vi "Set Time Context.vi"(0 "Tree in":refnum<class "Tree.lvclass">, 5 "Start":refnum<class "Data.lvclass">, 7 "End":refnum<class "Data.lvclass">, 9 "Delta":refnum<class "Data.lvclass">, 11 "error in (no error)":errorcluster) -> (4 "Tree out":refnum<class "Tree.lvclass">, 15 "error out":errorcluster)   [LabVIEW 2012, in "MDSplus.lvlib" / "Tree.lvclass"]
doc: "Set the current time context. Only the specified portion of segmented data will be returned by TreeNode.getData() method."
uses:
  <vilib>/MDSplus/Classes/Tree_Class/Tree.lvclass
  <vilib>/MDSplus/Classes/Data_Class/Data.lvclass
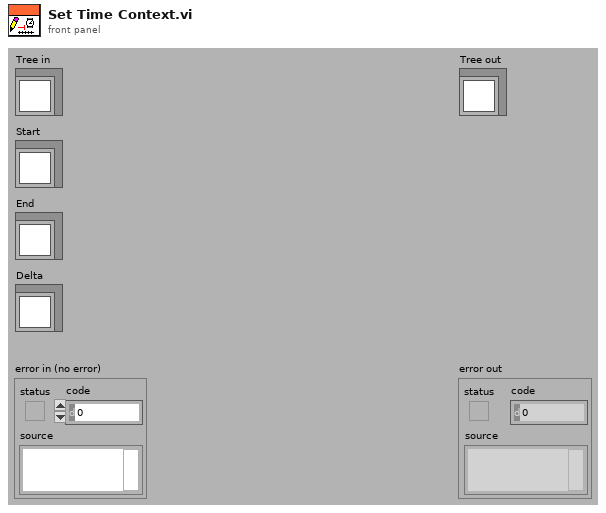
[diagram p1: front panel]
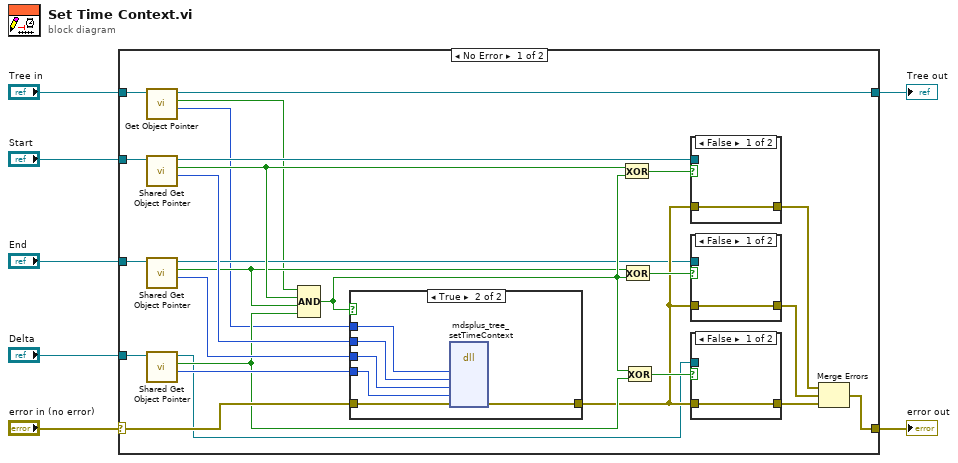
[diagram p0: block diagram]
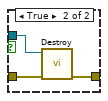
[diagram p2: hidden frame]
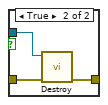
[diagram p3: hidden frame]
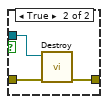
[diagram p4: hidden frame]
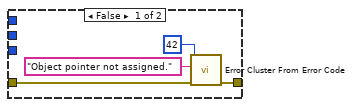
[diagram p5: hidden frame]
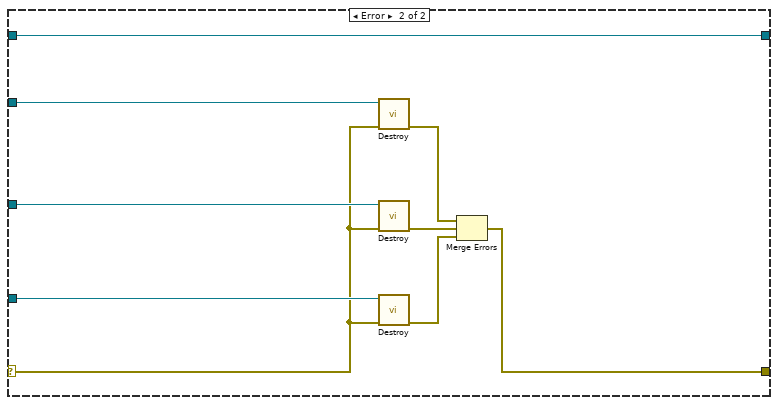
[diagram p6: hidden frame]
diagram:
  n1 = case shown="No Error" "error in (no error)" {
    selector: "error in (no error)" -> [w27 w57]
    tunnel: [w12 w56] -> w6
    tunnel: [w10 w64] -> w5
    tunnel: "Tree in" -> [w11 w64]
    tunnel: "Start" -> [w33 w63]
    tunnel: "End" -> [w32 w62]
    tunnel: "Delta" -> [w31 w61]
    frame No Error {
      n2 = call-dynamic "Get Object Pointer.vi"("Tree in"=w11) -> ("Object Pointer"=w9:i64, "Assigned object pointer?"=w8:bool, "Tree out"=w10:refnum<class "Tree.lvclass">)  [unwired: 8 in]
      n3 = call <vilib>:"Shared Get Object Pointer.vi"("Data in"=w33) -> ("Object Pointer"=w28:i64, "Assigned object pointer?"=w23:bool, "Data out"=w18:refnum<class "Data.lvclass">)  [unwired: 8 in]
      n4 = call <vilib>:"Shared Get Object Pointer.vi"("Data in"=w32) -> ("Object Pointer"=w29:i64, "Assigned object pointer?"=w20:bool, "Data out"=w17:refnum<class "Data.lvclass">)  [unwired: 8 in]
      n5 = call <vilib>:"Shared Get Object Pointer.vi"("Data in"=w31) -> ("Object Pointer"=w30:i64, "Assigned object pointer?"=w22:bool, "Data out"=w16:refnum<class "Data.lvclass">)  [unwired: 8 in]
      n6 = Compound Arithmetic op=AND(w8, w23, w20, w22) -> (w21:bool)
      n7 = case shown="True" w21 {
        tunnel: w30 -> [_ w55]
        tunnel: w29 -> [_ w54]
        tunnel: w28 -> [_ w53]
        tunnel: w27 -> [w47 w52]
        tunnel: [w46 w51] -> w19
        tunnel: w9 -> [_ w50]
        frame False {
          n8 = call <vilib>:"Error Cluster From Error Code.vi"("error in (no error)"=w47, "error message (\"\")"="Object pointer not assigned." ("error message (\"\")"), "error code (0)"=42) -> ("error out"=w46:errorcluster)  [unwired: 6 in]
        }
        frame True {
          n9 = dll-call lib="MDSobjectsLVShr" fn="mdsplus_tree_setTimeContext"("lvTreePtr"=w50, "lvStartDataPtrIn"=w53, "lvEndDataPtrIn"=w54, "lvDeltaDataPtrIn"=w55, "error"=w52) -> ("error"=w51:errorcluster)  [unwired: 8 in, 2 out]
        }
      }
      n10 = Exclusive Or(1:w21, 2:w23) -> (0:w26:bool)
      n11 = Exclusive Or(1:w21, 2:w20) -> (0:w25:bool)
      n12 = Exclusive Or(1:w22, 2:w21) -> (0:w24:bool)
      n13 = case shown="False" w26 {
        tunnel: w19 -> [w38 w41]
        tunnel: w18 -> [_ w40]
        tunnel: [w38 w39] -> w13
        frame False {
        }
        frame True {
          n14 = call-dynamic "Destroy.vi"("error in (no error)"=w41, "Data in"=w40) -> ("error out"=w39:errorcluster)  [unwired: 9 in]
        }
      }
      n15 = case shown="False" w25 {
        tunnel: w19 -> [w42 w45]
        tunnel: w17 -> [_ w44]
        tunnel: [w42 w43] -> w14
        frame False {
        }
        frame True {
          n16 = call-dynamic "Destroy.vi"("error in (no error)"=w45, "Data in"=w44) -> ("error out"=w43:errorcluster)  [unwired: 9 in]
        }
      }
      n17 = case shown="False" w24 {
        tunnel: w19 -> [w34 w37]
        tunnel: w16 -> [_ w36]
        tunnel: [w34 w35] -> w15
        frame False {
        }
        frame True {
          n18 = call-dynamic "Destroy.vi"("error in (no error)"=w37, "Data in"=w36) -> ("error out"=w35:errorcluster)  [unwired: 9 in]
        }
      }
      n19 = Merge Errors(w13, w14, w15) -> (w12:errorcluster)
    }
    frame Error {
      n20 = call-dynamic "Destroy.vi"("error in (no error)"=w57, "Data in"=w63) -> ("error out"=w58:errorcluster)  [unwired: 9 in]
      n21 = call-dynamic "Destroy.vi"("error in (no error)"=w57, "Data in"=w62) -> ("error out"=w60:errorcluster)  [unwired: 9 in]
      n22 = call-dynamic "Destroy.vi"("error in (no error)"=w57, "Data in"=w61) -> ("error out"=w59:errorcluster)  [unwired: 9 in]
      n23 = Merge Errors(w58, w60, w59) -> (w56:errorcluster)
    }
  }
  "error out" <- w6
  "Tree out" <- w5
